vi "DataLog Read Chunk By Index.vi"(0 "tag log directory":path, 1 "index in last chunk":i32, 5 "index of last chunk":i32, 11 "error in (no error)":errorcluster, 12 "chunk index":i32) -> (4 "dup tag log directory":path, 6 "last chunk in log?":bool, 8 "chunk of points":T1[](array[typedef]) {"value" format="%.3e"; "time" format="%<%H:%M:%S%2u\n%Y/%m/%d>T"}, 15 "error out":errorcluster)   [LabVIEW 2012]
doc: "Read the chunk with the given index from the log. When the last chunk in the log is requested, only as many points as present will be returned."
uses:
  typedefs/clusters/t_DataLog Point.ctl
  glb_DataLog MCVD.vi
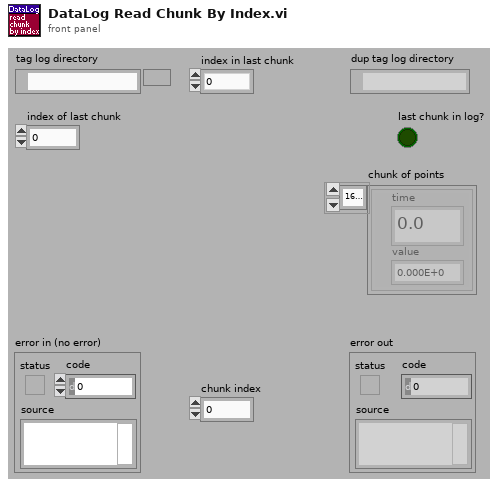
[diagram p1: front panel]
types:
  T1 = typedef "t_DataLog Point.ctl" = cluster{"time":dbl, "value":dbl}
  T2 = enum16{"read/write", "read-only", "write-only", "write-only (truncate)"}
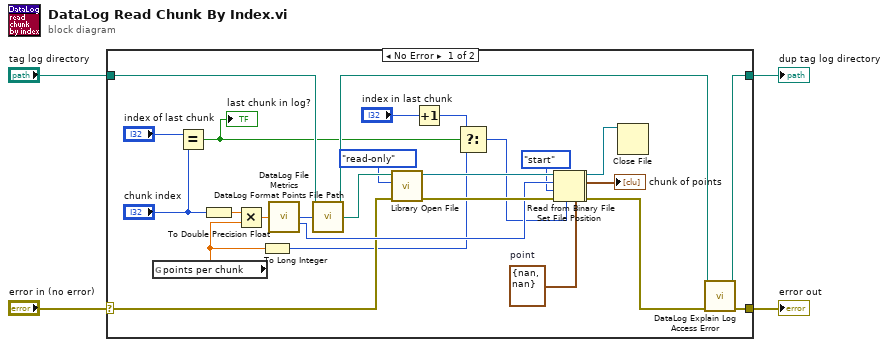
[diagram p0: block diagram]
diagram:
  n1 = case shown="No Error" "error in (no error)" {
    selector: "error in (no error)" -> [w18 w34]
    tunnel: [w20 w34] -> w4
    tunnel: "tag log directory" -> [w17 w33]
    tunnel: [w19 w33] -> w1
    frame No Error {
      w13 = T1 {"time"=nan, "value"=nan}  # point
      n2 = global read "glb_DataLog MCVD.vi" "points per chunk"() -> (w26:dbl)
      n3 = Equal?(x="index of last chunk", y="chunk index") -> (x = y?=w10:bool)
      "last chunk in log?" <- w10
      n4 = To Double Precision Float(number="chunk index") -> (double precision float=w25:dbl)
      n5 = Multiply(x=w25, y=w26) -> (x*y=w24:dbl)
      n6 = To Long Integer(number=w26) -> (32bit integer=w8:i32)
      n7 = call "DataLog File Metrics.vi"("point index"=w24) -> ("log file index"=w23:i32, "log file offset"=w22:i32)  [unwired: 9 in, 4 out]
      n8 = call "DataLog Format Points File Path.vi"("tag log directory"=w17, "log file index"=w23) -> ("dup tag log directory"=w16:path, "log file path"=w32:path)  [unwired: 12 in]
      n9 = call "Library Open File.vi"("error in (no error)"=w18, "open mode (read/write)"=T2."read-only" ("open mode (0)"), "file path"=w32) -> ("error out"=w29:errorcluster, "refnum"=w30:refnum<file>)  [unwired: 3 in]
      n10 = Increment(x="index in last chunk") -> (x+1=w9:i32)
      n11 = Select(t=w9, s=w10, f=w8) -> (s? t:f=w7:i32)
      n12 = Set File Position(offset (in bytes) (0)=w22, refnum=w30, from (0:start)=enum16{"start", "end", "current"}."start" ("pos mode (0:2)"), error in=w29) -> (refnum out=w6:refnum<file>, error out=w5:errorcluster)
      n13 = Read from Binary File(5:w13, 8:w5, 10:w7, 11:w6) -> (0:w21:errorcluster, 2:→"chunk of points":T1[], 3:w31:refnum<file>)  [unwired: 2 in, 1 out]
      n14 = Close File(refnum=w31) -> ()  [unwired: 1 in, 2 out]
      n15 = call "DataLog Explain Log Access Error.vi"("tag log directory"=w16, "error in"=w21) -> ("dup tag log directory"=w19:path, "error out"=w20:errorcluster)  [unwired: 12 in]
    }
    frame Error {
    }
  }
  "error out" <- w4
  "dup tag log directory" <- w1
